vi "Find Raw Zero.vi"(1 "steeringPower":dbl[](array[numeric])) -> (0 "powerOutput":dbl[](array[numeric]))   [LabVIEW 2019]
uses:
  swerveData.vi
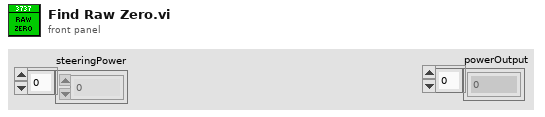
[diagram p1: front panel]
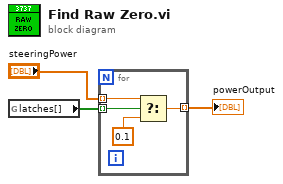
[diagram p0: block diagram]
diagram:
  n1 = global read "swerveData.vi" "latches[]"() -> (w1:bool[])
  n2 = for {
    tunnel: w1 -> [w6] mode=indexing
    tunnel: [w5] -> w2 mode=indexing
    tunnel: "steeringPower" -> [w4] mode=indexing
    n3 = Select(t=w4, s=w6, f=0.1) -> (s? t:f=w5:dbl)
  }
  "powerOutput" <- w2
